vi "AnalysatorNameInListeFinden.vi"(10 "AnalysatorDefinition":T1, 11 "AnalysatorListe":T1[](array[typedef])) -> (0 "Analysator":T1, 1 "gefunden":bool, 2 "Index":i32, 3 "AnalysatorListe out":T1[](array[typedef]))   [LabVIEW 2020, in "System Einstellungen V2.lvlib"]
uses:
  System Einstellungen V2.lvlib
  AnalysatorDefinition.ctl
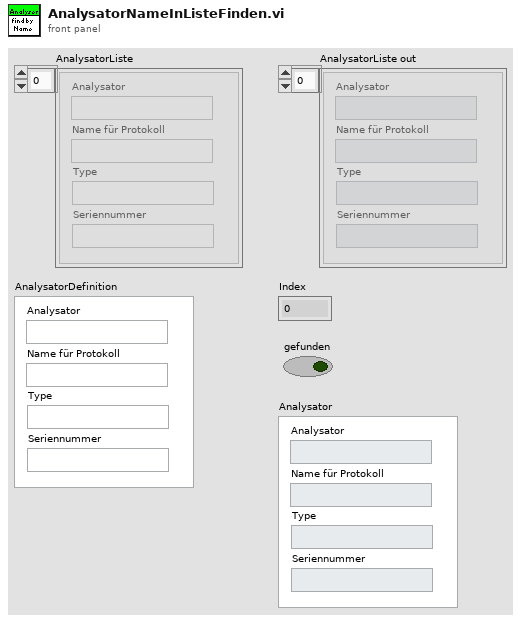
[diagram p1: front panel]
types:
  T1 = typedef "System Einstellungen V2.lvlib/AnalysatorDefinition.ctl" = cluster{"Analysator":string, "Name für Protokoll":string, "Type":string, "Seriennummer":string}
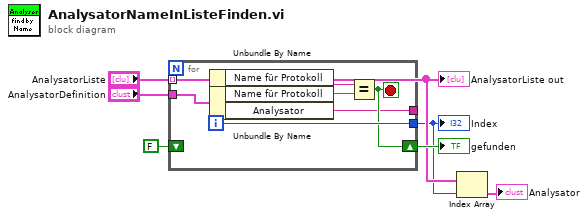
[diagram p0: block diagram]
diagram:
  n1 = for {
    tunnel: "AnalysatorDefinition" -> [w12]
    tunnel: "AnalysatorListe" -> [w13] mode=indexing
    tunnel: [w9] -> w2
    shift-right: [w8] -> w4
    shift-left: FALSE -> [_]
    tunnel: [w7] -> _
    i -> [w9]
    stop <- w8 stop-if-true
    n2 = Unbundle By Name(w13) -> ("Name für Protokoll"=w11:string)
    n3 = Unbundle By Name(w12) -> ("Name für Protokoll"=w10:string, "Analysator"=w7:string)
    n4 = Equal?(x=w11, y=w10) -> (x = y?=w8:bool)
  }
  "Index" <- w2
  "gefunden" <- w4
  n5 = Index Array(array="AnalysatorListe", index=w2) -> (element=→"Analysator":T1)
  "AnalysatorListe out" <- "AnalysatorListe"
